vi "Read - Fetch IQ Data.vi"(0 "session in":T1[](array[typedef]) {"rx baseband session"."3630 session"."Address Space" items=["VXI/VME A16"=1, "VXI/VME A24"=2, "VXI/VME A32"=3, "VXI/VME A64"=4, "PXI Memory Allocations"=9, "PXI Configuration"=10, "PXI BAR0"=11, "PXI BAR1"=12, "PXI BAR2"=13, "PXI BAR3"=14, "PXI BAR4"=15, "PXI BAR5"=16]; "tx baseband session"."3610 session"."Address Space" items=["VXI/VME A16"=1, "VXI/VME A24"=2, "VXI/VME A32"=3, "VXI/VME A64"=4, "PXI Memory Allocations"=9, "PXI Configuration"=10, "PXI BAR0"=11, "PXI BAR1"=12, "PXI BAR2"=13, "PXI BAR3"=14, "PXI BAR4"=15, "PXI BAR5"=16]}, 7 "number of samples":u32=8192, 11 "error in":errorcluster, 12 "Timeout (ms)":i32=5000) -> (4 "session out":T1[](array[typedef]) {"rx baseband session"."3630 session"."Address Space" items=["VXI/VME A16"=1, "VXI/VME A24"=2, "VXI/VME A32"=3, "VXI/VME A64"=4, "PXI Memory Allocations"=9, "PXI Configuration"=10, "PXI BAR0"=11, "PXI BAR1"=12, "PXI BAR2"=13, "PXI BAR3"=14, "PXI BAR4"=15, "PXI BAR5"=16]; "tx baseband session"."3610 session"."Address Space" items=["VXI/VME A16"=1, "VXI/VME A24"=2, "VXI/VME A32"=3, "VXI/VME A64"=4, "PXI Memory Allocations"=9, "PXI Configuration"=10, "PXI BAR0"=11, "PXI BAR1"=12, "PXI BAR2"=13, "PXI BAR3"=14, "PXI BAR4"=15, "PXI BAR5"=16]}, 8 "data [channel]":cluster{"data":i16[]}[](array[cluster]), 15 "error out":errorcluster)   [LabVIEW 2019, in "mmWave HW Control.lvlib"]
uses:
  mmWave HW Control.lvlib
  Low-level/TypeDefs/Session.ctl
  <instrlib>/niMmWave/ni3620/Config/v1/Host/Public/High-Level/niMmWave Session.ctl
  <instrlib>/_niInstr/Register Bus/v0/Host/Public/Register Bus Session.ctl
  <instrlib>/_niInstr/Register Bus/v0/Host/Private/Session Data.ctl
  <instrlib>/niMmWave/ni3620/Config/v1/Host/Public/Typedefs/Board Information.ctl
  <instrlib>/niMmWave/ni3620/Config/v1/Host/Public/Typedefs/Hardware Revision.ctl
  <instrlib>/niMmWave/ni3620/Config/v1/Host/Public/Typedefs/Gain Mapping.ctl
  <instrlib>/niMmWave/ni3620/Config/v1/Host/Public/Typedefs/Correction Data.ctl
  <instrlib>/niMmWave/ni3620/Config/v1/Host/Public/Typedefs/Opera Characterization.ctl
  <instrlib>/niMmWave/ni3620/Config/v1/Host/Public/Corrections/Typedefs/Opera Characterization Main Header.ctl
  <instrlib>/niMmWave/ni3620/Config/v1/Host/Public/Corrections/Typedefs/Opera IF Board Information.ctl
  <instrlib>/niMmWave/ni3620/Config/v1/Host/Public/Corrections/Typedefs/Opera Characterization Instance Header.ctl
  <instrlib>/niMmWave/ni3620/Config/v1/Host/Public/Corrections/Typedefs/Opera Characterization Device Data Header.ctl
  <instrlib>/niMmWave/ni3620/Config/v1/Host/Public/Corrections/Typedefs/Opera LO Characterization Data Header.ctl
  <instrlib>/niMmWave/ni3620/Config/v1/Host/Public/Corrections/Typedefs/Opera IF Board Characterization Data Header.ctl
  <instrlib>/niMmWave/ni3620/Config/v1/Host/Public/Corrections/Typedefs/Opera Characterization Device Data.ctl
  <instrlib>/niMmWave/ni3620/Config/v1/Host/Public/Corrections/Typedefs/Opera LO2 Board Characterization Data.ctl
  <instrlib>/niMmWave/ni3620/Config/v1/Host/Public/Corrections/Typedefs/Opera LO Characterization Data.ctl
  <instrlib>/niMmWave/ni3620/Config/v1/Host/Public/Corrections/Typedefs/Opera IF Board Characterization Data.ctl
  <instrlib>/niMmWave/ni3620/Config/v1/Host/Public/Corrections/Typedefs/Opera IQ Impairment Data.ctl
  <instrlib>/niMmWave/ni3620/Config/v1/Host/Public/Typedefs/mmWave Adapter Session Data.ctl
  <instrlib>/niMmWave/ni3620/Config/v1/Host/Public/Typedefs/mmWave Adapter Data.ctl
  <instrlib>/niMmWave/ni3620/Config/v1/Host/Public/Typedefs/mmWave Adapter 2.ctl
  <instrlib>/niMmWave/ni3620/Config/v1/Shared/Typedefs/Subsystem ID.ctl
  <instrlib>/niMmWave/ni3620/Config/v1/Host/Public/Typedefs/mmWave Adapter Channel Information.ctl
  <instrlib>/niMmWave/ni3620/Config/v1/Host/Public/Typedefs/Temperature Coefficients.ctl
  <instrlib>/niMmWave/ni3620/Config/v1/Host/Public/Typedefs/mmWave Characterization.ctl
  <instrlib>/niMmWave/ni3620/Config/v1/Host/Public/Corrections/Typedefs/mmWave Characterization Main Header.ctl
  <instrlib>/niMmWave/ni3620/Config/v1/Host/Public/Corrections/Typedefs/mmWave Characterization Instance Header.ctl
  <instrlib>/niMmWave/ni3620/Config/v1/Host/Public/Typedefs/Session Cache.ctl
  <instrlib>/niMmWave/ni3620/Config/v1/Host/Public/Typedefs/LO2 settings cache.ctl
  <instrlib>/niMmWave/ni3620/Config/v1/Host/Public/Typedefs/LO2 source.ctl
  <instrlib>/niMmWave/ni3620/Config/v1/Host/Public/Typedefs/Desired and Coerced.ctl
  <instrlib>/niMmWave/ni3620/Config/v1/Host/Public/Typedefs/Export cache.ctl
  <instrlib>/niMmWave/ni3620/Config/v1/Host/Public/Typedefs/Path cache.ctl
  <instrlib>/niMmWave/ni3620/Config/v1/Host/Public/Typedefs/Daughterboard Type.ctl
  <instrlib>/niMmWave/ni3620/Config/v1/Host/Public/Typedefs/LO1 settings cache.ctl
  <instrlib>/niMmWave/ni3620/Config/v1/Host/Public/Typedefs/LO1 Source.ctl
  <instrlib>/niMmWave/ni3620/Config/v1/Host/Public/Typedefs/mmWave export cache.ctl
  <instrlib>/niMmWave/ni3620/Config/v1/Host/Private/Board/LO2/LO2 Board Configuration Cache.ctl
  <instrlib>/niMmWave/ni3620/Config/v1/Host/Public/Typedefs/reference clock routing settings.ctl
  <instrlib>/niMmWave/ni3620/Config/v1/Host/Public/Typedefs/LO2 routing settings.ctl
  <instrlib>/niMmWave/ni3620/Config/v1/Host/Private/Board/LO1/LO1 Board Configuration Cache.ctl
  <instrlib>/niMmWave/ni3620/Config/v1/Host/Public/Typedefs/LO1 source settings.ctl
  <instrlib>/niMmWave/ni3620/Config/v1/Host/Public/Typedefs/LO1 export settings.ctl
  <instrlib>/niMmWave/ni3620/Config/v1/Host/Public/Typedefs/LO1 mmWave settings.ctl
  Low-level/TypeDefs/Tx Baseband Session.ctl
  <instrlib>/niMmWave/ni3610 and ni3630/controls/public/Main Settings.ctl
  <vilib>/Instr/_visa.llb/VISA Register Access Address Space.ctl
  <instrlib>/niMmWave/ni3610 and ni3630/controls/public/Register Adresses.ctl
  <instrlib>/niMmWave/ni3610 and ni3630/controls/public/Base Card Type.ctl
  <instrlib>/niMmWave/ni3610 and ni3630/controls/private/IQ Card Revision.ctl
  <instrlib>/niMmWave/ni3610 and ni3630/controls/public/Board Capability.ctl
  Low-level/TypeDefs/Blank FPGA Reference.ctl
  Low-level/TypeDefs/Rx Baseband Session.ctl
  Low-level/TypeDefs/Hardware Configuration.ctl
  Low-level/TypeDefs/Direction.ctl
  Low-level/TypeDefs/Gain Ranging.ctl
  Low-level/TypeDefs/PXI Trigger Bus Info.ctl
  Low-level/TypeDefs/RX driver FPGA ref.ctl
  <vilib>/Utility/error.llb/Error Cluster From Error Code.vi
  <vilib>/rvi/errors/niLvFpgaAdjustHostInterfaceError.vi
  <vilib>/rvi/interface/nirviMethod/nirviMethod.xnode
  <vilib>/FPGAPlugInAG/Dynamic/niLvFpga_ReadFifo_Dynamic.vi
  <vilib>/rvi/errors/niLvFpgaMergeErrorWithErrorCode.vi
  <instrlib>/_niInstr/Register Bus/v0/Host/niInstr Register Bus v0 Host.lvlib
  <instrlib>/niMmWave/ni3610 and ni3630/ni3610_and_ni3630_Driver_Lib.lvlib
  <instrlib>/niMmWave/ni3620/Config/v1/Host/niMmWave Config v1 Host.lvlib
  <instrlib>/niMmWave/ni3620/Config/v1/Shared/niMmWave Config v1 Shared.lvlib
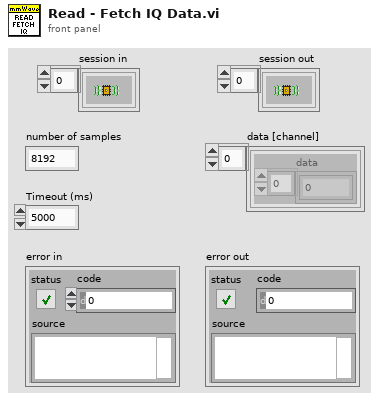
[diagram p1: front panel]
types:
  T1 = typedef "Session.ctl" = cluster{"3620 session":refnum<queue>, "tx baseband session":T2, "rx baseband session":T10, "tx gain (dB)":dbl, "rx gain (dB)":dbl, "hardware configuration":T11, "gain ranging":T13[], "pxi trigger bus information":T14}
  T2 = typedef "Tx Baseband Session.ctl" = cluster{"3610 session":T3, "7902 reference":T9}
  T3 = typedef "ni3610_and_ni3630_Driver_Lib.lvlib/Main Settings.ctl" = cluster{"VISA resource name":refnum<visa-resource-name>, "Address Space":T4, "window_offset":u32, "register_addresses":T5, "required_MM_fpga_version":cluster{"signature":u32, "hardware":u32, "current revision":u32, "oldest revision":u32}, "CPLD Oldest Compat Version ":cluster{"hardware":u32, "CPLD firmware":u32}, "MM_FPGA_image_location":string, "is_init":bool, "card_type":T6, "DacLmkConfigFileName":string, "AdcLmkConfigFileName":string, "AdcConfigFileName":string, "DacConfigFileName_RevA":string, "DacConfigFileName_RevB":string, "Mulde hardware revision":u8, "bypass DAC PLL\n":bool, "IQ Card Revision":T7, "board capability":T8}
  T4 = typedef "VISA Register Access Address Space.ctl" = u16
  T5 = typedef "ni3610_and_ni3630_Driver_Lib.lvlib/Register Adresses.ctl" = cluster{"MM based Registers":cluster{"Revision":u32, "OldestCompatRev":u32, "signature":u32, "scratch":u32, "LedControl":u32, "BoardHwRev":u32, "BoardControl":u32, "ThermalStatus":u32, "BasebandStatus":u32, "BasebandControl":u32, "BasebandAuxSetup":u32, "BasebandAuxStatus":u32, "LmkSyncOutSetup":u32, " AdcSyncOutSetup":u32, " InjSyncOutSetup":u32, " PxiTrig0OutSetup":u32, " PxiTrig1OutSetup":u32, " PxiTrig2OutSetup":u32, " PxiTrig3OutSetup":u32, " PxiTrig4OutSetup":u32, " PxiTrig5OutSetup":u32, " PxiTrig6OutSetup":u32, " PxiTrig7OutSetup":u32}, "CPLD based Registers":cluster{"SlaveSignature":u32, "SlaveRevision":u32, "SlaveOldestCompatRev":u32, "SlaveScratch":u32, "SlaveSetup":u32, "SlaveStatus":u32, "IDacReg_offset":u32, "LMKRegGrp0_offset":u32, "QDacReg_offset":u32, "BrdTempSensorVal":u32, "TempSensorPowerDown":u32, "GPIOReg_offset":u32, "IAdcReg_offset":u32, "QAdcReg_offset":u32, "LMKRegGrp1_offset":u32, "QadcTempSensorVal":u32, "IadcTempSensorVal":u32, "RevisionReg":u32, "VcxoReg":u32, "CpldStatusReg":u32, "PowerReg":u32, "VBiasEnReg":u32, "ExtRefOeReg":u32, "QdacCtrlReg":u32, "QdacStatusReg":u32, "IdacCtrlReg":u32, "IdacStatusReg":u32, "QdacJtagIn":u32, "QdacJtagOut":u32, "IdacJtagIn":u32, "IdacJtagOut":u32, "IqDcSetupReg":u32, "QadcStatusReg":u32, "IadcStatusReg":u32, "BrdSetupReg":u32, "IqDcRevisionReg":u32, "PllStatusReg":u32, "EndpointScratchReg":u32, "AdcSyncCfgReg":u32, "IqCardOpampReg":u32}, "CPLD Register Offset":u32, "MM  Register Offset":u32, " PxiTrig0OutSetup":u32}
  T6 = typedef "ni3610_and_ni3630_Driver_Lib.lvlib/Base Card Type.ctl" = enum16{"unspecified", "ADC", "DAC"}
  T7 = typedef "ni3610_and_ni3630_Driver_Lib.lvlib/IQ Card Revision.ctl" = enum16{"RevA", "RevB", "RevC", "RevD"}
  T8 = typedef "ni3610_and_ni3630_Driver_Lib.lvlib/Board Capability.ctl" = cluster{"baseband sync":enum16{"no baseband sync", "baseband sync"}}
  T9 = typedef "Blank FPGA Reference.ctl" = refnum<k20>
  T10 = typedef "Rx Baseband Session.ctl" = cluster{"3630 session":T3, "7902 reference":T9}
  T11 = typedef "Hardware Configuration.ctl" = cluster{"direction":T12, "baseband only":bool}
  T12 = typedef "Direction.ctl" = enum16{"Transceiver", "Receiver", "Transmitter"}
  T13 = typedef "Gain Ranging.ctl" = cluster{"gain ranging active scope":string, "gain ranging stream session":refnum<k20>}
  T14 = typedef "PXI Trigger Bus Info.ctl" = cluster{"chassis resource name":refnum<visa-resource-name>, "7902R (TX)":i16, "3610 (TX)":i16, "3620 (IF)":i16, "3630 (RX)":i16, "7902R (RX)":i16}
  T15 = typedef "RX driver FPGA ref.ctl" = refnum<k20>
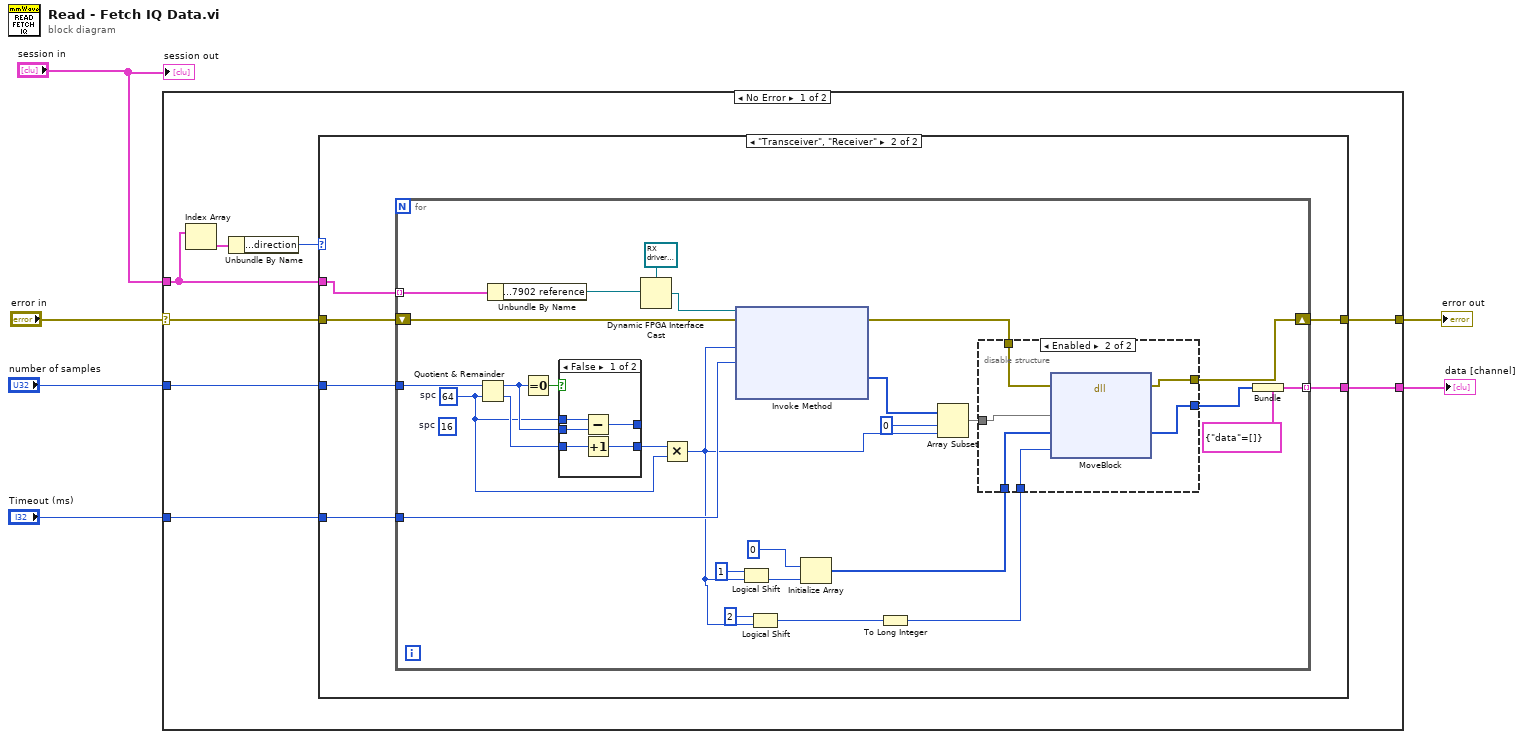
[diagram p0: block diagram]
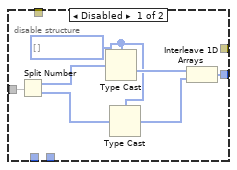
[diagram p3: hidden frame]
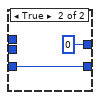
[diagram p4: hidden frame]
diagram:
  n1 = case shown="No Error" "error in" {
    selector: "error in" -> [w14 w70]
    tunnel: [w12 w70] -> w5
    tunnel: "session in" -> [w10 _]
    tunnel: "number of samples" -> [w13 _]
    tunnel: [w11 _] -> w2
    tunnel: "Timeout (ms)" -> [w7 _]
    frame No Error {
      n2 = Index Array(array=w10) -> (element=w9:T1)  [unwired: 1 in]
      n3 = Unbundle By Name(w9) -> ("hardware configuration.direction"=w8:T12)
      n4 = case shown="\"Transceiver\", \"Receiver\"" w8 {
        tunnel: w14 -> [w15 w21]
        tunnel: w10 -> [_ w17]
        tunnel: w13 -> [_ w20]
        tunnel: [w15 w19] -> w12
        tunnel: [_ w18] -> w11
        tunnel: w7 -> [_ w16]
        frame "Transmitter" {
        }
        frame "Transceiver", "Receiver" {
          n5 = for {
            tunnel: w20 -> [w48]
            shift-right: [w22] -> w19
            shift-left: w21 -> [w49]
            tunnel: [w40] -> w18 mode=indexing
            tunnel: w17 -> [w39] mode=indexing
            tunnel: w16 -> [w35]
            (unwired) u32 16  # spc
            w33 = u32 64  # spc
            n6 = Quotient & Remainder(x=w48, y=w33) -> (x-y*floor(x/y)=w44:u32, floor(x/y)=w45:u32)
            n7 = Unbundle By Name(w39) -> ("rx baseband session.7902 reference"=w37:T9)
            n8 = Equal To 0?(x=w44) -> (x = 0?=w46:bool)
            n9 = case shown="False" w46 {
              tunnel: w45 -> [w67 w69]
              tunnel: w44 -> [w65 _]
              tunnel: [w66 w69] -> w43
              tunnel: w33 -> [w64 _]
              tunnel: [w63 u64 0] -> _
              frame False {
                n10 = Subtract(x=w64, y=w65) -> (x-y=w63:u32)
                n11 = Increment(x=w67) -> (x+1=w66:u32)
              }
              frame True {
              }
            }
            n12 = Dynamic FPGA Interface Cast(Session In=T15 refnum ("Type"), Type=w37) -> (Session Out=w36:T15)
            n13 = Multiply(x=w43, y=w33) -> (x*y=w28:u32)
            n14 = xnode "Invoke Method"("FPGA VI Reference In"=w36, "error in"=w49, "Number of Elements"=w28, "Timeout (ms)"=w35) -> ("error out"=w23:errorcluster, "Data"=w47:u32[])  [unwired: 2 out]
            n15 = Logical Shift(y=i16 1, x=w28) -> (x << y=w30:u32)
            n16 = Logical Shift(y=i16 2, x=w28) -> (x << y=w25:u32)
            n17 = Initialize Array(i16 0, w30) -> (w26:i16[])
            n18 = To Long Integer(number=w25) -> (32bit integer=w24:i32)
            n19 = Array Subset(array=w47, index=0, length=w28) -> (w42:u32[])
            n20 = disable-structure shown="Enabled" {
              disable-tunnel: w42 -> [w56 w61]
              disable-tunnel: [w54 w60] -> w32
              disable-tunnel: w26 -> [_ w62]
              disable-tunnel: w24 -> [_ w59]
              disable-tunnel: w23 -> [_ w58]
              disable-tunnel: [_ w57] -> w22
              frame Disabled {
                w51 = i16[] [] ("data")
                n21 = Split Number(x=w56) -> (hi(x)=w55:u16[], lo(x)=w52:u16[])
                n22 = Type Cast(type=w51, x=w55) -> (*(type *) &x=w53:i16[])
                n23 = Type Cast(type=w51, x=w52) -> (*(type *) &x=w50:i16[])
                n24 = Interleave 1D Arrays(w53, w50) -> (w54:i16[])
              }
              frame Enabled {
                n25 = dll-call lib="LabVIEW" fn="MoveBlock"(error in=w58, "psrc"=w61, "pdst"=w62, "size"=w59) -> (error out=w57:errorcluster, "pdst"=w60:i16[])  [unwired: 5 in, 1 out]
              }
            }
            n26 = Bundle(cluster=cluster{"data":i16[]} {"data"=[]} ("data"), "data"=w32) -> (w40:cluster{"data":i16[]})
          }
        }
      }
    }
    frame Error {
    }
  }
  "error out" <- w5
  "data [channel]" <- w2
  "session out" <- "session in"
